vi "Create Publish Config URL.vi"(6 "Group (All)":string, 9 "port":i32, 10 "ip":u32) -> (2 "String":string)   [LabVIEW 2020, in "Vecto.lvlib"]
uses:
  Vecto.lvlib
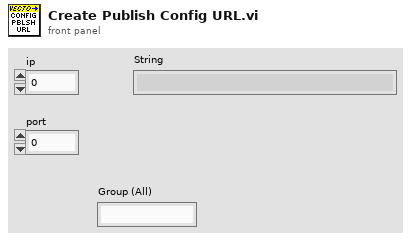
[diagram p1: front panel]
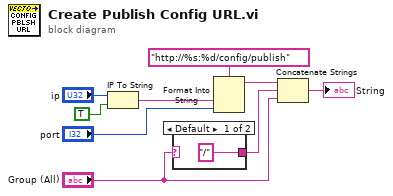
[diagram p0: block diagram]
diagram:
  n1 = IP To String(1:TRUE ("dot notation? (F)"), 2:"ip") -> (0:w6:string)
  n2 = case shown="Default" "Group (All)" {
    selector: "Group (All)" -> [_ w11]
    tunnel: ["/" w11] -> w2
    frame Default {
    }
    frame "" {
    }
  }
  n3 = Format Into String(format string="http://%s:%d/config/publish", w6, "port") -> (resulting string=w4:string)  [unwired: 2 in, 1 out]
  n4 = Concatenate Strings(w4, w2, "Group (All)") -> (→"String":string)
